vi "SEW_Modbus_Velocity.vi"(0 "Remote IP Address":string="127.0.0.1", 1 "Timeout [ms]":u32=10000, 3 "Output (Write Multiple Register) 2":u16[](array[numeric]) format="%x") -> (5 "Input (Read Holding Register) 2":u16[](array[numeric]) format="%04x")   [LabVIEW 2023]
uses:
  <vilib>/Plasmionique/MB Master/MB_Master_TCP/MB_Master_TCP.lvclass
  <vilib>/Plasmionique/MB Master/MB Master.lvlib
panel:
  out "error out 2":errorcluster caption="error out"
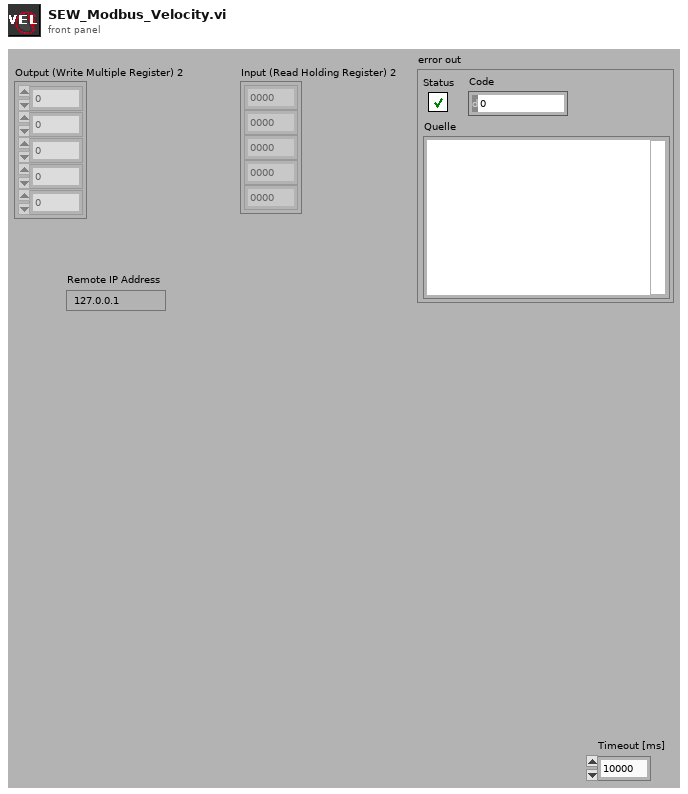
[diagram p1: front panel]
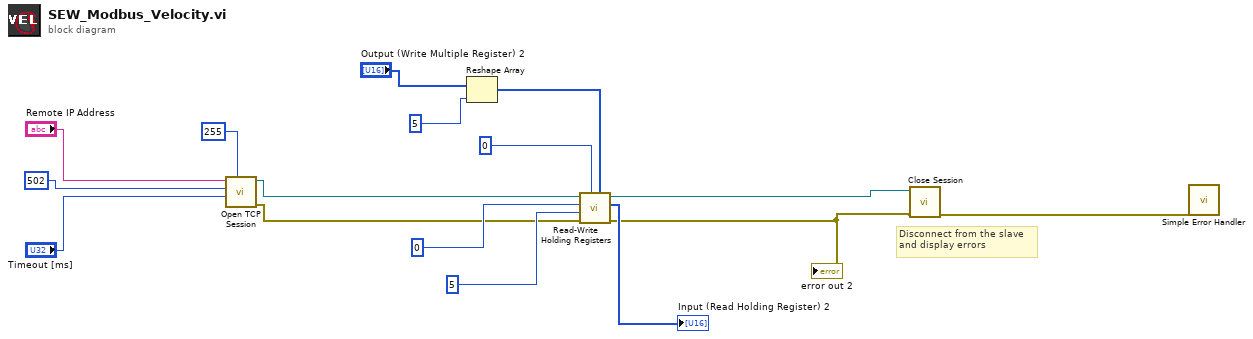
[diagram p0: block diagram]
diagram:
  # "Disconnect from the slave\nand display errors"
  n1 = call <vilib>:"Open TCP Session.vi"("Slave ID (255)"=u16 255 ("Remote Port"), "Timeout (10000)"="Timeout [ms]", "Port (502)"=u16 502 ("Remote Port"), "IP Address"="Remote IP Address") -> ("error out"=w3:errorcluster, "MB_TCP session"=w4:refnum<class "MB_Master_TCP.lvclass">)  [unwired: 6 in]
  n2 = Reshape Array("Output (Write Multiple Register) 2", 5) -> (w6:u16[])
  n3 = call <vilib>:"Read-Write Holding Registers.vi"("write values"=w6, "write starting address"=u16 0 ("Remote Port"), "error in (no error)"=w3, "read quantity"=u16 5 ("Remote Port"), "read starting address"=u16 0 ("Remote Port"), "MB session in"=w4) -> ("error out"=w1:errorcluster, "read registers"=→"Input (Read Holding Register) 2":u16[], "MB session out"=w2:refnum<class "MB_Master_TCP.lvclass">)  [unwired: 3 in]
  "error out 2" <- w1
  n4 = call-dynamic "Close Session.vi"("error in (no error)"=w1, "MB TCP session"=w2) -> ("error out"=w12:errorcluster)  [unwired: 9 in]
  n5 = call <vilib>:"Simple Error Handler.vi"("error in (no error)"=w12) -> ()  [unwired: 1 in, 8 out]
